vi "BI.vi"(1 "Ctl Refnum 2":refnum<vi>, 2 "Ctl Refnum":refnum<vi>, 8 "error in (no error)":errorcluster caption="错误输入（无错误）", 9 "客户仪器地址":refnum<visa-resource-name>="USB0::0x0471::0x2826::QF71600867::INSTR", 10 "Cluster 2":cluster{"文本路径：":path, "表格路径：":path}={"文本路径："=path "C:/Users/shipeng/Desktop/BIAS Dielectric measurement Log", "表格路径："=path "C:/Users/shipeng/Desktop/BIAS Dielectric measurement Log"}, 11 "起始偏压":dbl[][](array[numeric])=[[-5.0, 5.0, 21.0], [5.0, -5.0, 21.0], [-5.0, 0.0, 10.0]]) -> (0 "错误输出":cluster{"状态":bool, "代码":i32, "源":string})   [LabVIEW 2017]
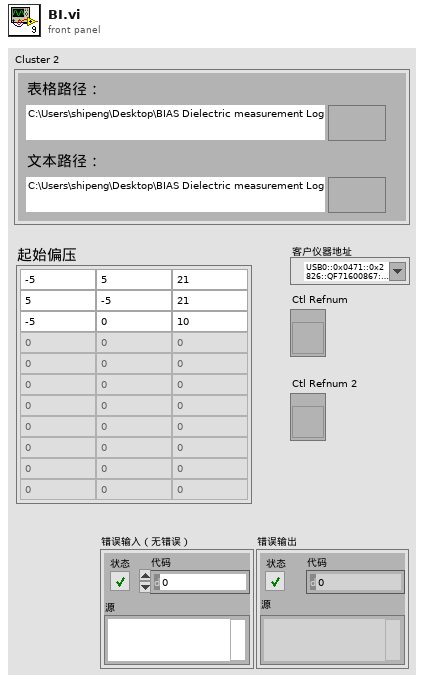
[diagram p1: front panel]
types:
  T1 = enum16{"open", "replace", "create", "open or create", "replace or create", "replace or create with confirmation"}
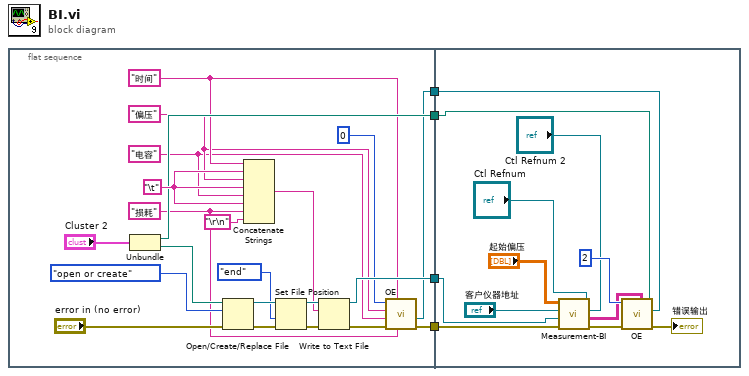
[diagram p0: block diagram]
diagram:
  n1 = flat-sequence {
    tunnel: [w17] -> w4
    tunnel: [w6] -> w3
    tunnel: [w13] -> w2
    tunnel: [w5] -> w1
    tunnel: w4 -> [w37]
    tunnel: w3 -> [w34]
    tunnel: w2 -> [w32]
    tunnel: w1 -> [w35]
    frame #0 {
      w8 = "损耗" ("字符串")
      w9 = "电容" ("字符串")
      w10 = "偏压" ("字符串")
      w18 = "\t"
      w11 = "时间" ("字符串")
      n2 = Unbundle("Cluster 2") -> ("文本路径："=w13:path, "表格路径："=w14:path)
      n3 = Open/Create/Replace File(file path (use dialog)=w14, error in="error in (no error)", operation (0:open)=T1."open or create" ("操作(0:open)")) -> (refnum out=w24:refnum<file>, error out=w21:errorcluster)  [unwired: 4 out]
      n4 = Concatenate Strings(w11, w18, w10, w18, w9, w18, w8, "\r\n") -> (w20:string)
      n5 = Set File Position(refnum=w24, from (0:start)=enum16{"start", "end", "current"}."end" ("自（0:起始）"), error in=w21) -> (refnum out=w25:refnum<file>, error out=w26:errorcluster)  [unwired: 1 out]
      n6 = Write to Text File(file (use dialog)=w25, text=w20, error in=w26) -> (refnum out=w17:refnum<file>, error out=w7:errorcluster)  [unwired: 2 out]
      n7 = call "OE.vi"("String 4"=w8, "String"=w11, "error in (no error)"=w7, "String 3"=w9, "String 2"=w10, "Numeric"=0) -> ("error out"=w5:errorcluster, "report out"=w6:refnum<class "NI_report.lvclass">)  [unwired: 3 in, 1 out]
    }
    frame #1 {
      n8 = call "Measurement-BI.vi"("Ctl Refnum 2"="Ctl Refnum 2", "Ctl Refnum"="Ctl Refnum", "error in (no error)"=w35, "Byte Stream File Refnum"=w37, "客户仪器地址"="客户仪器地址", "起始偏压"="起始偏压") -> ("error out"=w30:errorcluster, "Array"=w31:string[][])  [unwired: 4 in]
      n9 = call "OE.vi"("report in"=w34, "表格数据路径："=w32, "Array"=w31, "error in (no error)"=w30, "Numeric"=2) -> ("error out"=→"错误输出":errorcluster)  [unwired: 4 in, 2 out]
    }
  }
